vi "K avg filter (using FIR vi).vi"(9 "avg num":i32=10, 11 "x":dbl format="%0.2f") -> (3 "Filtered x":dbl format="%0.2f")   [LabVIEW 2018]
uses:
  <vilib>/ptbypt/NI_PtbyPt.lvlib
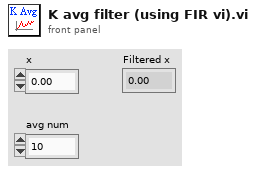
[diagram p1: front panel]
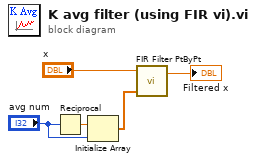
[diagram p0: block diagram]
diagram:
  n1 = Reciprocal(x="avg num") -> (1/x=w5:dbl)
  n2 = Initialize Array(w5, "avg num") -> (w4:dbl[])
  n3 = call <vilib>:"FIR Filter PtByPt.vi"("Forward Coefficients"=w4, "x"="x") -> ("Filtered x"=→"Filtered x":dbl)  [unwired: 2 in, 1 out]
